vi "GlobalStop.vi"(0 "Set":bool, 5 "Reset":bool) -> (4 "Stop":bool)   [LabVIEW 2019]
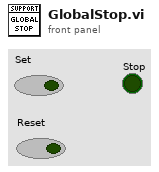
[diagram p1: front panel]
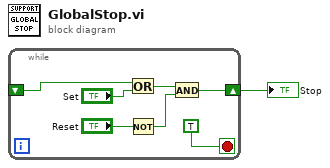
[diagram p0: block diagram]
diagram:
  n1 = while {
    shift-right: [w6] -> w1
    shift-left: _ -> [w3]
    stop <- TRUE stop-if-true
    n2 = Or(x=w3, y="Set") -> (x .or. y?=w7:bool)
    n3 = Not(x="Reset") -> (.not. x?=w4:bool)
    n4 = And(x=w7, y=w4) -> (x .and. y?=w6:bool)
  }
  "Stop" <- w1
